vi "AlliGator SS3 Gates Slip Correction.vi"(8 "error in (no error)":errorcluster, 11 "Data Value Reference in":refnum<data-value>) -> (0 "error out":errorcluster, 1 "Message":string, 3 "Data Value Reference out":refnum<data-value>)   [LabVIEW 2021, in "AlliGator HDF5.lvlib"]
doc: "Performs the column truncation for SS3 datasets needed to fix a common FPGA data transfer issue."
uses:
  AlliGator HDF5.lvlib
  Internal Variables/AlliGator Internal Variables v2.ctl
  <vilib>/vision/Image Controls.llb/IMAQ Image.ctl
  Internal Variables/AlliGator Gate Image Set.ctl
  Files/AlliGator FLI Dataset Type.ctl
  Files/AlliGator Data Series Type.ctl
  Dual-Channel Datasets/AlliGator Dataset Channel.ctl
  Settings/AlliGator Gate Arithmetic.ctl
  Source Image/AlliGator Displayed Image.ctl
  Image/Named ROI Description.ctl
  Phasor Graph/AlliGator Decay Metadata v3.ctl
  Decay Analysis/Decay Preprocessing/AlliGator Decay Background Subtraction Info.ctl
  Decay Analysis/Decay Preprocessing/AlliGator Baseline Subtraction Method.ctl
  Graphs/XY Graph/XY Graph Plot Shift Parameters.ctl
  Graphs/XY Graph/XY Graph Plot Shift Method.ctl
  Decay Analysis/Decay Preprocessing/AlliGator Decay Extrapolation Parameters.ctl
  Phasor/Calibration Phasor (m, phi).ctl
  Phasor/Phasor Reference Series.ctl
  Phasor/Phasor Calibration Map v2.ctl
  Phasor/Phasor (g, s).ctl
  Phasor Graph/AlliGator Raw Phasor Plot Data v5.ctl
  Phasor/Phasor Standard Deviation Options.ctl
  Phasor Plot/AlliGator Phasor Multi-Harmonic Data.ctl
  Phasor/Phasor Harmonic Data.ctl
  Decay Fit Parameter Map/AlliGator Decay Fit Options & Parameters v4.ctl
  Fits/IRF(X)PSED/Decay Fit Options v4.ctl
  Fits/Decay Convolution/Decay Model.ctl
  Fits/Residual Type.ctl
  Fits/IRF(X)PSED/Fit Weights Type v2.ctl
  Fits/Non-linear Fitting Method v2.ctl
  Fits/Fit Calculation Method.ctl
  Fits/Non-linear Fitting Algorithm.ctl
  Decay Analysis/Decay Fit/AlliGator Decay Fit Parameter Constraints 2.ctl
  Fits/IRF(X)PSED/Decay Fit Parameters In List.ctl
  Fits/IRF(X)PSED/MLE Baseline Offset Type.ctl
  Decay Analysis/Decay Preprocessing/AlliGator Decay Preprocessing Parameters.ctl
  Fits/IRF(X)PSED/Decay Fit Parameters & Derived Quantities List v2.ctl
  Fits/IRF(X)PSED/Decay Fit Result Constraint.ctl
  Decay Fit Parameter Map/AlliGator Parameter Maps Data.ctl
  Files/AlliGator Files.lvlib
  <vilib>/vision/NI_Vision_Development_Module.lvlib
  Phasor/Phasor.lvlib
  Image/Image.lvlib
  Decay Analysis/Decay Preprocessing/AlliGator Decay Preprocessing.lvlib
  Graphs/XY Graph/XY Graph Add-Ons.lvlib
  Phasor Graph/AlliGator Phasor Graph.lvlib
  Phasor Plot/AlliGator Phasor Plot.lvlib
  Source Image/AlliGator Source Image.lvlib
  Fits/Fits.lvlib
  Internal Variables/AlliGator Internal Variables.lvlib
  Decay Analysis/Decay Fit/AlliGator Decay Fit.lvlib
  Settings/AlliGator Settings.lvlib
  Dual-Channel Datasets/AlliGator Dual-Channel Datasets.lvlib
  Decay Fit Parameter Map/AlliGator Decay Fit Parameter Map.lvlib
panel:
  # "see the AlliGator License on the block diagram (Ctrl+E or Window:Show Block Diagram)"
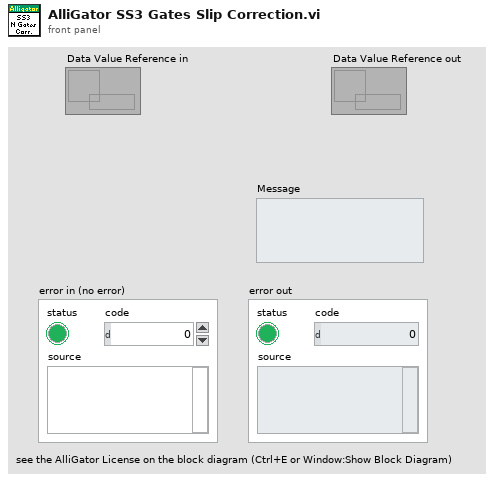
[diagram p1: front panel]
types:
  T1 = typedef "IMAQ Image.ctl" = refnum<image>
  T2 = typedef "AlliGator Internal Variables.lvlib/AlliGator Internal Variables v2.ctl" = cluster{"----------------------------- Images -----------------------------":u8, "Displayed Image":T1, "White Light Image":T1, "Mask Image":T1, "ROI Mask Image":T1, "Current Dataset Images 1":T3, "Background Dataset Images 1":T3, "Current Dataset Images 2":T3, "Background Dataset Images 2":T3, "Current Dataset Arithmetic Images":T3, "Accumulated Dataset Images 1":T3, "Accumulated Dataset Images 2":T3, "Accumulated Dataset Arithmetic Images":T3, "----------------------------- File Paths -----------------------------":u8, "Phasor Plot Image":T1, "Decay Fit Parameter Map Image":T1, "Parameter Map Image":T1, "Single Data Point Path":path, "White Light Image Path":path, "Mask Image Path":path, "Time-Series Folder":path, "[Time-Series Paths]":path[], "----------------------------- FLI Dataset -----------------------------":u8, "Current Dataset":i32, "Single Dataset Type":T4, "Current Folder":string, "AlliGator Data Series Type":T5, "# Datasets":i32, "Dual-Channel Dataset":bool, "Selected Channel Name":string, "Dataset Channel":T6, "Channel Arithmetic":T7, "Dual-Channel Background Dataset":bool, "Background Channel":T6, "Dual-Channel Accumulated Dataset":bool, "Start Time":dbl, "[Time-Series Timestamps]":dbl[], "[Intensity Corrections]":dbl[], "Time Series Script":bool, "Type of Displayed Image":T8, "Gate Image Slide":u16, "# Gates":i32, "ROIs":T9[], "----------------------------- Decays -----------------------------":u8, "ROI Decay":cluster{"t Array":dbl[], "I Array":dbl[]}, "Valid Decay":bool, "Decay  Metadata":T11, "Reference Decay Plot Name":string, "Reference Decay":cluster{"t Array":dbl[], "I Array":dbl[]}, "Decay Shift Plot":cluster{"Time Stamps":dbl[], "Decay Shifts":dbl[]}, "[Decays Max Values]":sgl[], "[Decays Min Values]":sgl[], "----------------------------- Calibration -----------------------------":u8, "Calibration Phasor":T17, "Calibration Phasor Series":T18, "Phasor Calibration Map":T19, "Calibration Map MD5 Digest":string, "----------------------------- Phasor Graph -----------------------------":u8, "Last Raw Phasor":T20, "Last Calibrated Phasor":T20, "Last Calibrated Phasor SDV":T20, "Phasor Graph:Phasor Plot":cluster{"g Array":dbl[], "s Array":dbl[]}, "Phasor Graph:Phasor SDV Plot":cluster{"g Array":dbl[], "s Array":dbl[]}, "[Phasor Graph:Raw Phasor Plots]":T21[], "Phasor Plot locked to Ref 1":i32, "[Phasor Plot(s) locked to Ref 1]":i32[], "[Phasor Plot(s) locked to Ref 2]":i32[], "[Pixel Phasors]":T20[], "----------------------------- Phasor Plot -----------------------------":u8, "[[Sum Image]]":dbl[][], "[[CSG Phasors]]":csg[][], "[[Valid Pixel?]]":bool[][], "[[Phasor Ratios]]":dbl[][], "[[Average Lifetimes]]":dbl[][], "Amplitude Weighted Average Lifetime":bool, "I/m/phi Dataset":cluster{"I/m/phi Dataset?":bool, "Base Frequency":dbl[unit], "Harmonic Orders":u8[]}, "Multi Phasor Plot Data":T23, "----------------------------- Decay Fit Parameter Map -----------------------------":u8, "Decay Fit Options & Parameters":T25, "Fit Options: Decay Preprocessing Parameters":T36, "Fit Options: Reference Decay":cluster{"t Array":dbl[], "I Array":dbl[]}, "Is Full Image Parameters Map":bool, "Is Single-Pixels Parameters Map":bool, "NLSF Parameters Map X Resolution":i32, "NLSF Parameters Map Y Resolution":i32, "[Single Decay Fit Parameters]":dbl[], "Fit Model":T27, "[[Multiple Decays Fit Parameters]]":dbl[][], "[[Multiple Decays Fit Parameter SDVs]]":dbl[][], "[[IRFs]]":dbl[][], "[ROI Descriptors]":T10[], "IRF Array Time Axis":dbl[], "Decay Array Time Axis":dbl[], "[Decay Fit Parameter Names]":T37[], "[Decay Sum]":dbl[], "Array of Decay Fit Result Constraints":T38[], "Selected ROIs Array":bool[], "----------------------------- Parameter Maps -----------------------------":u8, "[Map Set Names]":string[], "[Parameter Maps]":T39[], "[[User-defined Quantities]]":dbl[][], "User-defined Quantity":string}
  T3 = typedef "AlliGator Internal Variables.lvlib/AlliGator Gate Image Set.ctl" = cluster{"SGL Gate Images":T1[], "SGL Sum Image":T1, "SGL Max Image":T1, "SGL Min Image":T1}
  T4 = typedef "AlliGator Files.lvlib/AlliGator FLI Dataset Type.ctl" = enum16{"HDF5 FLI Dataset", "Gate Image Folder", ".sdt FLI Dataset (Becker & Hickl)", ".ptu FLI Dataset (PicoQuant)", "SS1 FLI Dataset", "SS2 FLI Dataset", "I/m/phi Dataset", ".bin FLI Dataset (PicoQuant Binned)", ".bin FLI Dataset (Piccolo Binned)", ".mat FLI Dataset"}
  T5 = typedef "AlliGator Files.lvlib/AlliGator Data Series Type.ctl" = enum16{"Not a Supported Series", "Gate Images Folder Series", "SwissSPAD 2 Dataset Series", "B&H FLI Dataset Series", "PicoQuant PTU FLI Dataset Series", "PicoQuant BIN FLI Dataset Series", "Piccolo hist BIN FLI Dataset Series", "HDF5 FLI Dataset Series"}
  T6 = typedef "AlliGator Dual-Channel Datasets.lvlib/AlliGator Dataset Channel.ctl" = enum16{"G2", "INT"}
  T7 = typedef "AlliGator Settings.lvlib/AlliGator Gate Arithmetic.ctl" = enum16{"None", "INT-G2", "G2/INT*<INT>", "(1 - G2/INT)*<INT>"}
  T8 = typedef "AlliGator Source Image.lvlib/AlliGator Displayed Image.ctl" = enum16{"Single Gate", "Sum of All Gates", "Max of All Gates", "Min of All Gates", "-", "White Ligth Image", "Mask Image"}
  T9 = typedef "Image.lvlib/Named ROI Description.ctl" = cluster{"ROI Descriptor":T10, "ROI Name":string, "Overlay Color":u32}
  T10 = typedef "ROI Descriptor" = cluster{"Global Rectangle":i32[], "Contours":cluster{"ID":enum32{"External", "Internal"}, "Type":u32, "Coordinates":i32[]}[]}
  T11 = typedef "AlliGator Phasor Graph.lvlib/AlliGator Decay Metadata v3.ctl" = cluster{"ROI Descriptor":T10, "ROI Center":cluster{"X":i32, "Y":i32}, "Decay Background Subtraction Info":T12, "Decay Reverted":bool, "Decay Smoothened":bool, "Decay Straightened":bool, "Fitted Tau (Decay Straightening)":dbl, "Decay Shift Parameters":T14, "Decay Shifted":bool, "Decay Extrapolated":bool, "Decay Extrapolation Parameters":T16, "Decay Normalized":bool, "Fold Decay":bool, "# Folds":u32}
  T12 = typedef "AlliGator Decay Preprocessing.lvlib/AlliGator Decay Background Subtraction Info.ctl" = cluster{"Laser Period":dbl[unit], "Gate Duration":dbl[unit], "Baseline Subtraction Method":T13, "Background Definition Range":cluster{"Min Gate":dbl[unit], "Max Gate":dbl[unit]}, "Total Intensity w/o Bkgd Subtraction":dbl, "Bkgd-subtracted Intensity (exp)":dbl, "# Data Points":i32, "Background/Gate":dbl, "Fitted Lifetime":dbl[unit], "Bkgd-subtracted Intensity (theo)":dbl}
  T13 = typedef "AlliGator Decay Preprocessing.lvlib/AlliGator Baseline Subtraction Method.ctl" = enum16{"Mean", "Min", "Square Gated Single-Exponential", "File", "Constant"}
  T14 = typedef "XY Graph Add-Ons.lvlib/XY Graph Plot Shift Parameters.ctl" = cluster{"Type":T15, "Shift":dbl[unit], "Threshold":dbl, "Rotate":bool}
  T15 = typedef "XY Graph Add-Ons.lvlib/XY Graph Plot Shift Method.ctl" = enum16{"Default", "CFD", "Threshold", "Cross-Correlation"}
  T16 = typedef "AlliGator Decay Preprocessing.lvlib/AlliGator Decay Extrapolation Parameters.ctl" = cluster{"Additional Points":u32, "Head Fraction":dbl, "Fitted Tau":dbl, "Use Periodicity":bool, "Use Cursors":bool, "Tail Fraction":dbl}
  T17 = typedef "Phasor.lvlib/Calibration Phasor (m, phi).ctl" = cluster{"m":dbl, "phi":dbl, "Phasor Frequency":dbl[unit], "Reference Lifetime":dbl[unit]}
  T18 = typedef "Phasor.lvlib/Phasor Reference Series.ctl" = cluster{"m Array":dbl[], "phi Array":dbl[], "Phasor Frequency":dbl[unit], "Calibration Lifetime":dbl[unit]}
  T19 = typedef "Phasor.lvlib/Phasor Calibration Map v2.ctl" = cluster{"Phasor Frequency":dbl[unit], "Calibration Lifetime":dbl[unit], "ROI Centers":cluster{"X":i32, "Y":i32}[], "ROI Descriptors":T10[], "Map Resolution X":i32, "Map Resolution Y":i32, "z Array":cdb[]}
  T20 = typedef "Phasor.lvlib/Phasor (g, s).ctl" = cluster{"g":dbl, "s":dbl}
  T21 = typedef "AlliGator Phasor Graph.lvlib/AlliGator Raw Phasor Plot Data v5.ctl" = cluster{"Phasor Plot Name":string, "Raw Phasor Plot":T20[], "Phasor Frequency":dbl[unit], "[Decay Metadata]":T11[], "Raw Phasor Plot SDV":T20[], "Phasor SDV Options":T22, "[Calibration Phasor]":T17[], "Intensity Array":dbl[]}
  T22 = typedef "Phasor.lvlib/Phasor Standard Deviation Options.ctl" = cluster{"Compute Estimated SDV":bool, "# Replicas":u32, "Use Estimated Average Phasor":bool}
  T23 = typedef "AlliGator Phasor Plot.lvlib/AlliGator Phasor Multi-Harmonic Data.ctl" = cluster{"Base Frequency":dbl[unit], "# Harmonics":u8, "Harmonic Orders":u8[], "Phasor Plot Settings Checksum":u64, "Phasor Harmonic Data Array":T24[]}
  T24 = typedef "Phasor.lvlib/Phasor Harmonic Data.ctl" = cluster{"Phasor Harmonic Name":string, "Phasor Plot Settings Checksum":u64, "Phasor Frequency":dbl[unit], "Base Frequency":dbl[unit], "Harmonic Order":u8, "Phasor Plot Parameters":string, "Phasor Array [[CSG]]":csg[][], "Dataset File Path":path}
  T25 = typedef "AlliGator Decay Fit Parameter Map.lvlib/AlliGator Decay Fit Options & Parameters v4.ctl" = cluster{"SYNC Period":dbl[unit], "Fit Options":T26, "Fit Parameter Constraints":T33[], "MLE Baseline Offset":dbl, "MLE Baseline Offset Type":T35}
  T26 = typedef "Fits.lvlib/Decay Fit Options v4.ctl" = cluster{"Show Fit Residuals":bool, "Fit Model":T27, "Residual Type":T28, "Max Decay Percentile":dbl, "Min Decay Percentile":dbl, "Show Full Decay":bool, "Weights":T29, "Fitting Method":T30, "Compute Parameter Uncertainties":bool, "Periodic Boundaries":bool, "Model Calculation":T31, "Period":dbl[unit], "Termination Criteria":cluster{"Max Iterations":i32, "Max Function Calls":i32, "Max Time":dbl[unit], "Function Tolerance":dbl, "Parameter Tolerance":dbl, "Gradient Tolerance":dbl, "Min Lambda":dbl, "Max Lambda":dbl, "Initial Tick Count":u32}, "Offset Resolution":dbl[unit], "Use Local IRF":bool, "Fitting Algorithm":T32, "Show Confidence Interval ":bool, "Confidence Level":dbl}
  T27 = typedef "Fits.lvlib/Decay Model.ctl" = enum16{"1-Exponential", "2-Exponentials"}
  T28 = typedef "Fits.lvlib/Residual Type.ctl" = enum16{"Standard", "Normalized", "Reduced"}
  T29 = typedef "Fits.lvlib/Fit Weights Type v2.ctl" = enum16{"Unweighted", "1/Variance (Neyman)", "1/Variance (Pearson)", "Best of All"}
  T30 = typedef "Fits.lvlib/Non-linear Fitting Method v2.ctl" = enum16{"Least Square", "Least Absolute Residual", "Bisquare", "MLE", "-", "Best of All"}
  T31 = typedef "Fits.lvlib/Fit Calculation Method.ctl" = enum16{"Simulation", "Convolution", "Integration"}
  T32 = typedef "Fits.lvlib/Non-linear Fitting Algorithm.ctl" = enum16{"Levenberg-Marquardt", "Trust-Region Dogleg"}
  T33 = typedef "AlliGator Decay Fit.lvlib/AlliGator Decay Fit Parameter Constraints 2.ctl" = cluster{"Fit Parameter":T34, "Min Value":dbl, "Max Value":dbl, "Global":bool, "Used":bool}
  T34 = typedef "Fits.lvlib/Decay Fit Parameters In List.ctl" = enum16{"Offset", "Baseline", "A_1", "tau_1", "A_2", "tau_2"}
  T35 = typedef "Fits.lvlib/MLE Baseline Offset Type.ctl" = enum32{"Absolute", "Percentage"}
  T36 = typedef "AlliGator Decay Preprocessing.lvlib/AlliGator Decay Preprocessing Parameters.ctl" = cluster{"Background Subtraction":bool, "Straighten Decay":bool, "Reverse Gates":bool, "1-Normalized Decay":bool, "Smoothen Decay":bool, "Smoothing Parameter":dbl, "Shift Decay":bool, "Decay Shift Parameters":T14, "Extrapolate Decay":bool, "Additional Points":u32, "Head Fraction":dbl, "Pixel-Normalize Decay":bool, "Use Periodicity":bool, "Use Cursors":bool, "Tail Fraction":dbl, "Use Decay Pre-Processing":bool, "Fold Decay":bool, "# Folds":u32, "[0-1]-Normalized Decay":bool}
  T37 = typedef "Fits.lvlib/Decay Fit Parameters & Derived Quantities List v2.ctl" = enum16{"Offset", "Baseline", "A_1", "tau_1", "A_2", "tau_2", "<tau>_a", "f1_a", "f2_a", "<tau>_i", "f1_i", "f2_i", "-", "R^2", "Chi^2"}
  T38 = typedef "Fits.lvlib/Decay Fit Result Constraint.ctl" = cluster{"Fit Parameter":enum16{"Offset", "Baseline", "A_1", "tau_1", "A_2", "tau_2", "<tau>_a", "f1_a", "f2_a", "<tau>_i", "f1_i", "f2_i", "-", "R^2", "Chi^2", "Max Relative Residual", "<Residual ACF>", "Residual ACF SDV", "tau_2/tau_1"}, "Min Value":dbl, "Max Value":dbl, "Use Constraint":bool}
  T39 = typedef "AlliGator Decay Fit Parameter Map.lvlib/AlliGator Parameter Maps Data.ctl" = cluster{"Map Set Name":string, "[Parameter Names]":string[], "[[Parameters]]":dbl[][], "[[Parameter SDVs]]":dbl[][], "Decay Array Time Axis":dbl[], "[[IRFs]]":dbl[][], "IRF Array Time Axis":dbl[], "X Resolution":i32, "Y Resolution":i32, "Intensity Array":dbl[]}
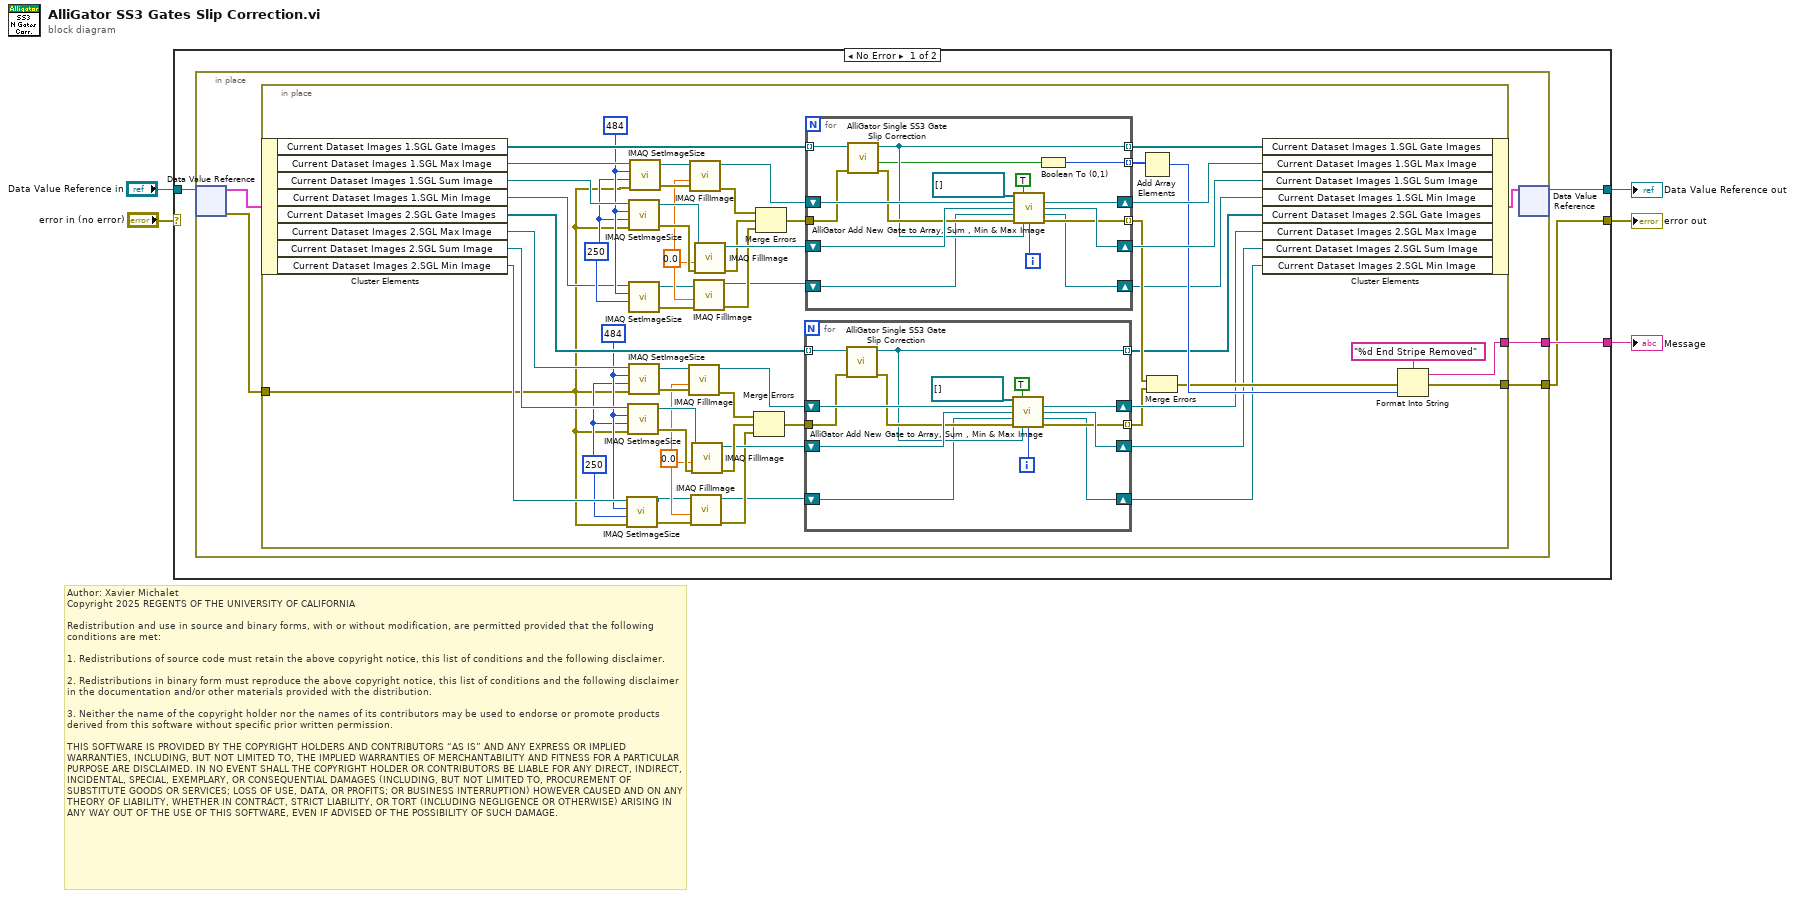
[diagram p0: block diagram]
diagram:
  # "Author: Xavier Michalet\nCopyright 2025 REGENTS OF THE UNIVERSITY OF CALIFORNIA\n\nRedistribution and use in source and binary forms, with or without modification, are permitted provided that the following conditions are met:\n\n1. Redistributions of source code must retain the above copyright notice, this list of conditions and the following disclaimer.\n\n2. Redistributions in binary form must reproduce the above copyright notice, this list of conditions and the following disclaimer in the documentation and/or other materials provided with the distribution.\n\n3. Neither the name of the copyright holder nor the names of its contributors may be used to endorse or promote products derived from this software without specific prior written permission.\n\nTHIS SOFTWARE IS PROVIDED BY THE COPYRIGHT HOLDERS AND CONTRIBUTORS “AS IS” AND ANY EXPRESS OR IMPLIED WARRANTIES, INCLUDING, BUT NOT LIMITED TO, THE IMPLIED WARRANTIES OF MERCHANTABILITY AND FITNESS FOR A PARTICULAR PURPOSE ARE DISCLAIMED. IN NO EVENT SHALL THE COPYRIGHT HOLDER OR CONTRIBUTORS BE LIABLE FOR ANY DIRECT, INDIRECT, INCIDENTAL, SPECIAL, EXEMPLARY, OR CONSEQUENTIAL DAMAGES (INCLUDING, BUT NOT LIMITED TO, PROCUREMENT OF SUBSTITUTE GOODS OR SERVICES; LOSS OF USE, DATA, OR PROFITS; OR BUSINESS INTERRUPTION) HOWEVER CAUSED AND ON ANY THEORY OF LIABILITY, WHETHER IN CONTRACT, STRICT LIABILITY, OR TORT (INCLUDING NEGLIGENCE OR OTHERWISE) ARISING IN ANY WAY OUT OF THE USE OF THIS SOFTWARE, EVEN IF ADVISED OF THE POSSIBILITY OF SUCH DAMAGE."
  n1 = case shown="No Error" "error in (no error)" {
    selector: "error in (no error)" -> [_ w103]
    tunnel: "Data Value Reference in" -> [w9 w102]
    tunnel: [w8 w102] -> w4
    tunnel: [w6 w103] -> w2
    tunnel: [w7 _] -> w1
    frame No Error {
      n2 = in-place {
        in-place-border: [w11] -> w7
        in-place-border: [w10] -> w6
        n3 = in-place-dvr #1(w9) -> (w14:T2, w12:errorcluster)
        n4 = in-place {
          in-place-border: w12 -> [w17]
          in-place-border: [w61] -> w11
          in-place-border: [w56] -> w10
          w18 = 250 ("Y Resolution")
          w19 = 484 ("X Resolution")
          w22 = sgl 0.0 ("Pixel Value (U8, U16, I16, Float)")
          w30 = 250 ("Y Resolution")
          w31 = 484 ("X Resolution")
          w32 = sgl 0.0 ("Pixel Value (U8, U16, I16, Float)")
          n5 = in-place-cluster #2(w14) -> ("Current Dataset Images 1.SGL Gate Images"=w71:T1[], "Current Dataset Images 1.SGL Max Image"=w55:T1, "Current Dataset Images 1.SGL Sum Image"=w54:T1, "Current Dataset Images 1.SGL Min Image"=w29:T1, "Current Dataset Images 2.SGL Gate Images"=w40:T1[], "Current Dataset Images 2.SGL Max Image"=w39:T1, "Current Dataset Images 2.SGL Sum Image"=w38:T1, "Current Dataset Images 2.SGL Min Image"=w20:T1)
          n6 = call "IMAQ SetImageSize"("error in (no error)"=w17, "Y Resolution"=w18, "X Resolution"=w19, "Image"=w20) -> ("error out"=w23:errorcluster, "Image Out"=w21:T1)  [unwired: 1 in]
          n7 = call "IMAQ SetImageSize"("error in (no error)"=w17, "Y Resolution"=w18, "X Resolution"=w19, "Image"=w38) -> ("error out"=w47:errorcluster, "Image Out"=w49:T1)  [unwired: 1 in]
          n8 = call "IMAQ SetImageSize"("error in (no error)"=w17, "Y Resolution"=w30, "X Resolution"=w31, "Image"=w54) -> ("error out"=w52:errorcluster, "Image Out"=w50:T1)  [unwired: 1 in]
          n9 = call "IMAQ SetImageSize"("Y Resolution"=w30, "X Resolution"=w31, "Image"=w29) -> ("error out"=w33:errorcluster, "Image Out"=w28:T1)  [unwired: 2 in]
          n10 = call "IMAQ SetImageSize"("error in (no error)"=w17, "Y Resolution"=w18, "X Resolution"=w19, "Image"=w39) -> ("error out"=w48:errorcluster, "Image Out"=w46:T1)  [unwired: 1 in]
          n11 = call "IMAQ SetImageSize"("error in (no error)"=w17, "Y Resolution"=w30, "X Resolution"=w31, "Image"=w55) -> ("error out"=w51:errorcluster, "Image Out"=w53:T1)  [unwired: 1 in]
          n12 = call "IMAQ FillImage"("error in (no error)"=w48, "Pixel Value (U8, U16, I16, Float)"=w22, "Image"=w46) -> ("error out"=w45:errorcluster, "Image Out"=w42:T1)  [unwired: 7 in]
          n13 = call "IMAQ FillImage"("error in (no error)"=w51, "Pixel Value (U8, U16, I16, Float)"=w32, "Image"=w53) -> ("error out"=w65:errorcluster, "Image Out"=w68:T1)  [unwired: 7 in]
          n14 = call "IMAQ FillImage"("error in (no error)"=w23, "Pixel Value (U8, U16, I16, Float)"=w22, "Image"=w21) -> ("error out"=w16:errorcluster, "Image Out"=w15:T1)  [unwired: 7 in]
          n15 = call "IMAQ FillImage"("error in (no error)"=w47, "Pixel Value (U8, U16, I16, Float)"=w22, "Image"=w49) -> ("error out"=w44:errorcluster, "Image Out"=w43:T1)  [unwired: 7 in]
          n16 = call "IMAQ FillImage"("error in (no error)"=w33, "Pixel Value (U8, U16, I16, Float)"=w32, "Image"=w28) -> ("error out"=w27:errorcluster, "Image Out"=w26:T1)  [unwired: 7 in]
          n17 = call "IMAQ FillImage"("error in (no error)"=w52, "Pixel Value (U8, U16, I16, Float)"=w32, "Image"=w50) -> ("error out"=w66:errorcluster, "Image Out"=w67:T1)  [unwired: 7 in]
          n18 = Merge Errors(w45, w44, w16) -> (w41:errorcluster)
          n19 = Merge Errors(w65, w66, w27) -> (w70:errorcluster)
          n20 = for {
            tunnel: w40 -> [w78] mode=indexing
            shift-right: [w81] -> w36
            shift-left: w42 -> [w83]
            shift-right: [w80] -> w35
            shift-left: w43 -> [w82]
            tunnel: w41 -> [w77]
            tunnel: [w79] -> w34 mode=indexing
            tunnel: [w75] -> w37 mode=indexing
            shift-right: [w73] -> w24
            shift-left: w15 -> [w72]
            i -> [w74]
            n21 = call "AlliGator Single SS3 Gate Slip Correction.vi"("error in (no error)"=w77, "Refnum in"=w78) -> ("error out"=w76:errorcluster, "Refnum out"=w75:T1)  [unwired: 7 in, 1 out]
            n22 = call "AlliGator Add New Gate to Array, Sum , Min & Max Image.vi"("SGL Gate Images in"=T1[] [], "Buffer Image Available"=TRUE, "SGL Image Max in"=w83, "SGL Image Sum in"=w82, "SGL Image Min in"=w72, "error in (no error)"=w76, "Gate Image"=w75, "Current Gate"=w74) -> ("SGL Image Max out"=w81:T1, "SGL Image Sum out"=w80:T1, "SGL Image Min out"=w73:T1, "error out"=w79:errorcluster)  [unwired: 3 in, 1 out]
          }
          n23 = for {
            tunnel: w71 -> [w94] mode=indexing
            shift-right: [w97] -> w64
            shift-left: w68 -> [w99]
            shift-right: [w96] -> w63
            shift-left: w67 -> [w98]
            tunnel: w70 -> [w93]
            tunnel: [w95] -> w60 mode=indexing
            tunnel: [w91] -> w69 mode=indexing
            tunnel: [w89] -> w62 mode=indexing
            shift-right: [w86] -> w25
            shift-left: w26 -> [w87]
            i -> [w88]
            n24 = call "AlliGator Single SS3 Gate Slip Correction.vi"("error in (no error)"=w93, "Refnum in"=w94) -> ("error out"=w92:errorcluster, "Last Strip Saturated?"=w90:bool, "Refnum out"=w91:T1)  [unwired: 7 in]
            n25 = call "AlliGator Add New Gate to Array, Sum , Min & Max Image.vi"("SGL Gate Images in"=T1[] [], "Buffer Image Available"=TRUE, "SGL Image Max in"=w99, "SGL Image Sum in"=w98, "SGL Image Min in"=w87, "error in (no error)"=w92, "Gate Image"=w91, "Current Gate"=w88) -> ("SGL Image Max out"=w97:T1, "SGL Image Sum out"=w96:T1, "SGL Image Min out"=w86:T1, "error out"=w95:errorcluster)  [unwired: 3 in, 1 out]
            n26 = Boolean To (0,1)(Boolean=w90) -> (0, 1=w89:i16)
          }
          n27 = Add Array Elements(numeric array=w62) -> (sum=w59:i16)
          n28 = Merge Errors(w60, w34) -> (w57:errorcluster)
          n29 = in-place-cluster #2("Current Dataset Images 1.SGL Gate Images"=w69, "Current Dataset Images 1.SGL Max Image"=w64, "Current Dataset Images 1.SGL Sum Image"=w63, "Current Dataset Images 1.SGL Min Image"=w25, "Current Dataset Images 2.SGL Gate Images"=w37, "Current Dataset Images 2.SGL Max Image"=w36, "Current Dataset Images 2.SGL Sum Image"=w35, "Current Dataset Images 2.SGL Min Image"=w24) -> (w13:T2)
          n30 = Format Into String(format string="%d End Stripe Removed", error in=w57, w59) -> (resulting string=w61:string, error out=w56:errorcluster)  [unwired: 1 in]
        }
        n31 = in-place-dvr #1(w13) -> (w8:refnum<data-value>)  [unwired: 1 out]
      }
    }
    frame Error {
    }
  }
  "error out" <- w2
  "Data Value Reference out" <- w4
  "Message" <- w1
